vi "Handle Debug Mode.vi"(8 "error in":errorcluster, 11 "path-with-auto-complete in":refnum<class "path-with-auto-complete.lvclass">) -> (0 "error out":errorcluster, 3 "path-with-auto-complete out":refnum<class "path-with-auto-complete.lvclass">)   [LabVIEW 2020, in "path-with-auto-complete.lvclass"]
uses:
  path-with-auto-complete.lvclass
  path-with-auto-complete.lvclass/path-with-auto-complete.ctl
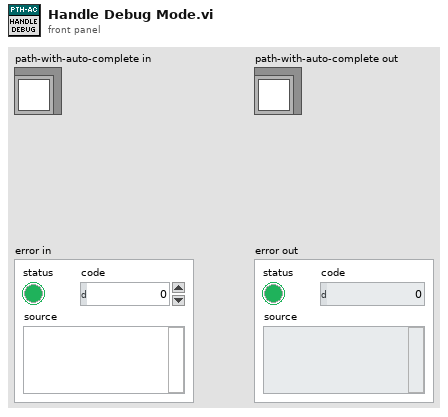
[diagram p1: front panel]
types:
  T1 = typedef "path-with-auto-complete.lvclass/State Data.ctl" = cluster{"Data":bool, "debug":bool, "mouse-down":bool, "has-focus":bool}
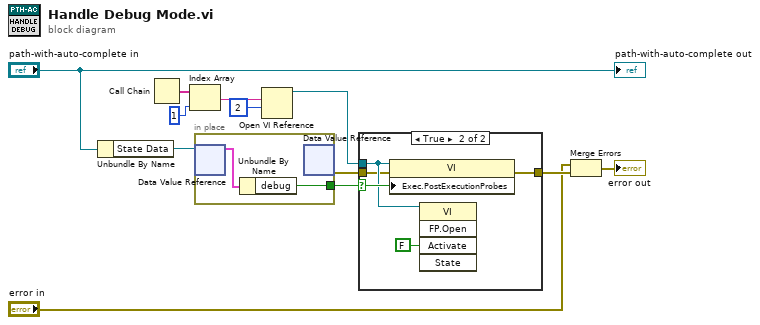
[diagram p0: block diagram]
diagram:
  n1 = Unbundle By Name("path-with-auto-complete in") -> ("State Data"=w11:refnum<data-value>)
  n2 = Call Chain() -> (call chain=w4:string[])
  n3 = Index Array(array=w4, index=1 ("Index")) -> (element=w6:string)
  n4 = in-place {
    in-place-border: [w14] -> w9
    n5 = in-place-dvr #1(w11) -> (w13:T1)  [unwired: 1 out]
    n6 = Unbundle By Name(w13) -> ("debug"=w14:bool)
    n7 = in-place-dvr #1() -> (w10:errorcluster)  [unwired: 1 in, 1 out]
  }
  n8 = Open VI Reference(vi path=w6, options=2) -> (vi reference=w3:refnum<vi>)  [unwired: 4 in, 1 out]
  n9 = case shown="True" w9 {
    selector: w9 -> [_ w20]
    tunnel: w3 -> [_ w19]
    tunnel: [w15 w17] -> w12
    tunnel: w10 -> [w15 w16]
    frame False {
    }
    frame True {
      n10 = property class="VI"(reference=w19, error in=w16, "Exec.PostExecutionProbes"=w20) -> (error out=w17:errorcluster)  [unwired: 1 out]
      n11 = invoke class="VI" method="FP.Open"(reference=w19, "Activate"=FALSE ("Activate?")) -> ()  [unwired: 3 in, 5 out]
    }
  }
  n12 = Merge Errors("error in", w12) -> (→"error out":errorcluster)
  "path-with-auto-complete out" <- "path-with-auto-complete in"
